vi "Fourier_Series_sagar.vi"() -> ()   [LabVIEW 2020]
panel:
  in  "stop":bool
  in  "Amplitude":dbl=0.7 format="%#_13g"
  in  "Frequency  (Hz)":i32=4000
  in  "Channel":i32(ring)=1 items=["Channel 1"=1, "Channel 2"=2]
  in  "Start":bool
  in  "Enum":enum16{"square", "saw"}(ring)=enum."saw"
  in  "Harmonics":i32
  out "Waveform Graph 1":dbl[](graph)
  in  "IP address":string="192.168.1.100"
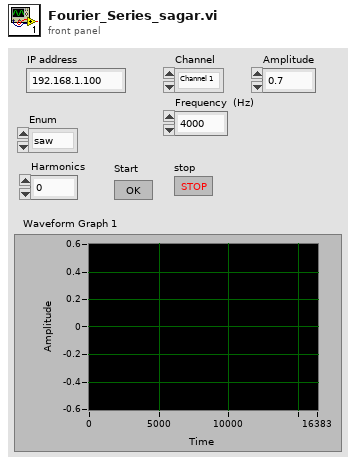
[diagram p1: front panel]
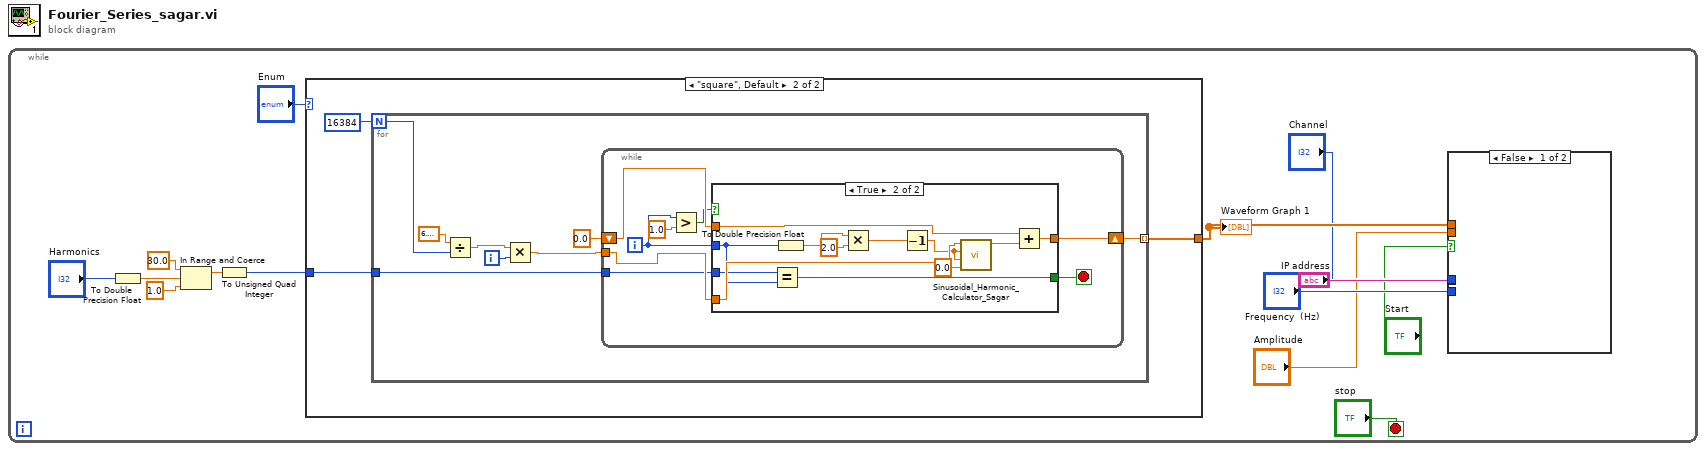
[diagram p0: block diagram]
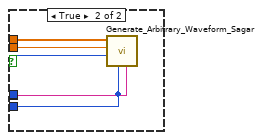
[diagram p2: hidden frame]
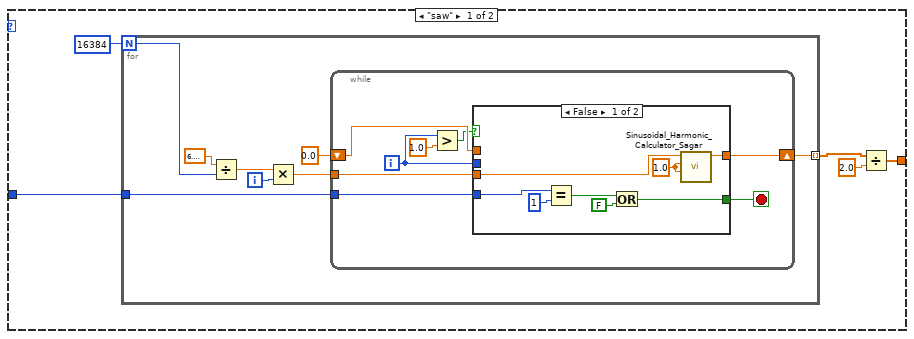
[diagram p3: hidden frame]
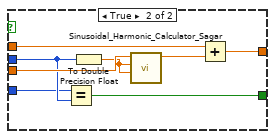
[diagram p4: hidden frame]
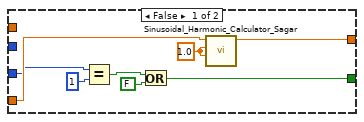
[diagram p5: hidden frame]
diagram:
  n1 = while {
    stop <- "stop" stop-if-true
    n2 = To Double Precision Float(number="Harmonics") -> (double precision float=w8:dbl)
    n3 = In Range and Coerce(upper limit=30.0, x=w8, lower limit=1.0) -> (coerced(x)=w11:dbl)  [unwired: 1 out]
    n4 = To Unsigned Quad Integer(1:w11) -> (0:w10:u64)
    n5 = case shown="\"square\", Default" "Enum" {
      tunnel: [w20 w58] -> w13
      tunnel: w10 -> [w23 w57]
      frame "saw" {
        n6 = for {
          N: 16384 -> [w31]
          tunnel: [w27] -> w21 mode=indexing
          tunnel: w23 -> [w25]
          i -> [w29]
          n7 = Divide(x=6.283185307179586, y=w31) -> (x/y=w30:dbl)
          n8 = Multiply(x=w30, y=w29) -> (x*y=w28:dbl)
          n9 = while {
            tunnel: w28 -> [w40]
            shift-right: [w37] -> w27
            shift-left: 0.0 -> [w38]
            tunnel: w25 -> [w33]
            i -> [w35]
            stop <- w39 stop-if-true
            n10 = Greater?(x=w35, y=1.0) -> (0:w34:bool)
            n11 = case shown="False" w34 {
              tunnel: w40 -> [w48 w56]
              tunnel: [w42 w55] -> w39
              tunnel: w38 -> [_ w54]
              tunnel: [w46 w52] -> w37
              tunnel: w35 -> [_ w51]
              tunnel: w33 -> [w41 w49]
              frame False {
                w47 = 1.0 ("Harmonic")
                n12 = Equal?(x=w41, y=1) -> (x = y?=w43:bool)
                n13 = Or(x=w43, y=FALSE) -> (x .or. y?=w42:bool)
                n14 = call "Sinusoidal_Harmonic_Calculator_Sagar.vi"("Amplitude (1/x)"=w47, "Harmonic"=w47, "Numeric in"=w48) -> ("Numeric out"=w46:dbl)  [unwired: 8 in]
              }
              frame True {
                n15 = Equal?(x=w49, y=w51) -> (x = y?=w55:bool)
                n16 = To Double Precision Float(number=w51) -> (double precision float=w50:dbl)
                n17 = call "Sinusoidal_Harmonic_Calculator_Sagar.vi"("Amplitude (1/x)"=w50, "Harmonic"=w50, "Numeric in"=w56) -> ("Numeric out"=w53:dbl)  [unwired: 8 in]
                n18 = Add(x=w54, y=w53) -> (x+y=w52:dbl)
              }
            }
          }
        }
        n19 = Divide(x=w21, y=2.0) -> (x/y=w20:dbl[])
      }
      frame "square", Default {
        n20 = for {
          N: 16384 -> [w66]
          tunnel: [w62] -> w58 mode=indexing
          tunnel: w57 -> [w60]
          i -> [w64]
          n21 = Divide(x=6.283185307179586, y=w66) -> (x/y=w65:dbl)
          n22 = Multiply(x=w65, y=w64) -> (x*y=w63:dbl)
          n23 = while {
            tunnel: w63 -> [w75]
            shift-right: [w72] -> w62
            shift-left: 0.0 -> [w73]
            tunnel: w60 -> [w68]
            i -> [w70]
            stop <- w74 stop-if-true
            n24 = Greater?(x=w70, y=1.0) -> (0:w69:bool)
            n25 = case shown="True" w69 {
              tunnel: w75 -> [w83 w95]
              tunnel: [w77 w94] -> w74
              tunnel: w73 -> [_ w93]
              tunnel: [w81 w91] -> w72
              tunnel: w70 -> [_ w86]
              tunnel: w68 -> [w76 w85]
              frame False {
                w82 = 1.0 ("Harmonic")
                n26 = Equal?(x=w76, y=1) -> (x = y?=w78:bool)
                n27 = Or(x=w78, y=FALSE) -> (x .or. y?=w77:bool)
                n28 = call "Sinusoidal_Harmonic_Calculator_Sagar.vi"("Amplitude (1/x)"=w82, "Harmonic"=w82, "Numeric in"=w83) -> ("Numeric out"=w81:dbl)  [unwired: 8 in]
              }
              frame True {
                n29 = Equal?(x=w85, y=w86) -> (x = y?=w94:bool)
                n30 = To Double Precision Float(number=w86) -> (double precision float=w87:dbl)
                n31 = Multiply(x=w87, y=2.0) -> (x*y=w89:dbl)
                n32 = Decrement(x=w89) -> (x-1=w88:dbl)
                n33 = call "Sinusoidal_Harmonic_Calculator_Sagar.vi"("Phase"=0.0, "Amplitude (1/x)"=w88, "Harmonic"=w88, "Numeric in"=w95) -> ("Numeric out"=w92:dbl)  [unwired: 7 in]
                n34 = Add(x=w93, y=w92) -> (x+y=w91:dbl)
              }
            }
          }
        }
      }
    }
    "Waveform Graph 1" <- w13
    n35 = case shown="False" "Start" {
      tunnel: w13 -> [_ w19]
      tunnel: "IP address" -> [_ w18]
      tunnel: "Channel" -> [_ w17]
      tunnel: "Frequency  (Hz)" -> [_ w16]
      tunnel: "Amplitude" -> [_ w15]
      frame False {
      }
      frame True {
        n36 = call "Generate_Arbitrary_Waveform_Sagar.vi"("Channel (1|2)"=w17, "IP address"=w18, "Frequency (1000 Hz)"=w16, "Channel (0: 1)"=w17, "Channel (1|2) 2"=w17, "Amplitude"=w15, "Array"=w19) -> ()  [unwired: 5 in]
      }
    }
  }
